vi "SMPS Inversion.vi"(8 "error in (no error)":errorcluster, 11 "DMA in":refnum<class "DMA.lvclass">) -> (0 "error out":errorcluster, 2 "IV Out":sgl[](array[numeric]), 3 "DMA out":refnum<class "DMA.lvclass">)   [LabVIEW 2014, in "DMA.lvclass"]
uses:
  DMA.lvclass
  DMA.lvclass/DMA.ctl
panel:
  out "Finished?":bool
  in  "smooth":u8
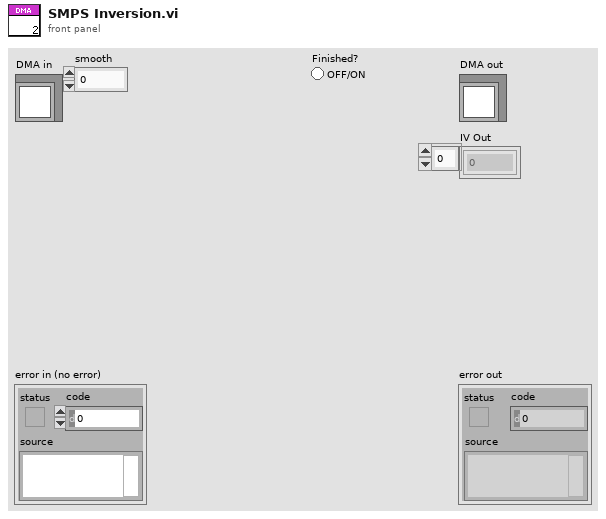
[diagram p1: front panel]
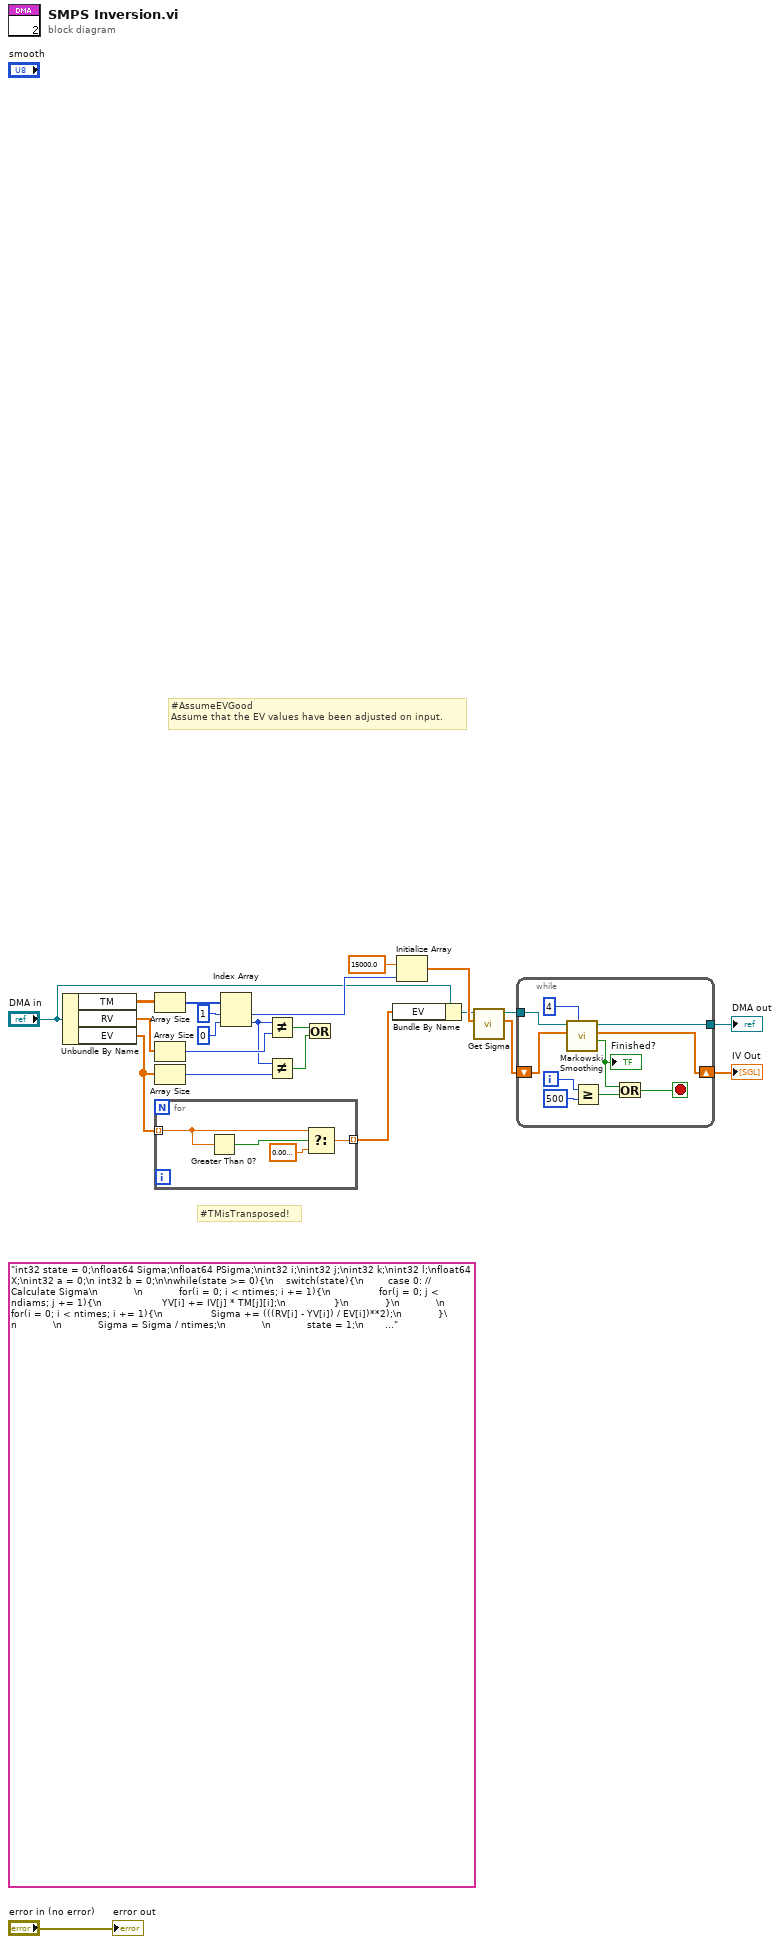
[diagram p0: block diagram]
diagram:
  (unwired) "int32 state = 0;\nfloat64 Sigma;\nfloat64 PSigma;\nint32 i;\nint32 j;\nint32 k;\nint32 l;\nfloat64 X;\nint32 a = 0;\n int32 b = 0;\n\nwhile(state >= 0){\n    switch(state){\n        case 0: // Calculate Sigma\n            \n            for(i = 0; i < ntimes; i += 1){\n                for(j = 0; j < ndiams; j += 1){\n                    YV[i] += IV[j] * TM[j][i];\n                }\n            }\n            \n            for(i = 0; i < ntimes; i += 1){\n                Sigma += (((RV[i] - YV[i]) / EV[i])**2);\n            }\n            \n            Sigma = Sigma / ntimes;\n            \n            state = 1;\n            \n    break;\n        case 1: // Twomey Iterations\n            \n            for(i = 0; i < ntimes; i += 1){\n                for(k = 0; k < ndiams; k += 1){\n                    X += TM[k][i] * IV[k];\n                }\n                X = RV[i] / X;\n                for(j = 0; j < ndiams; j += 1){\n                    IV[j] = (1 + (X - 1) * TM[j][i]) * IV[j];\n                }\n            }\n            \n            PSigma = Sigma;\n\n            for(i = 0; i < ntimes; i += 1){\n                for(j = 0; j < ndiams; j += 1){\n                    YV[i] += IV[j] * TM[j][i];\n                }\n            }\n            \n            for(i = 0; i < ntimes; i += 1){\n                Sigma += (((RV[i] - YV[i]) / EV[i])**2);\n            }\n            \n            Sigma = Sigma / ntimes;\n\n            a += 1;\n            \n            if(a >= 100){state = 2;}\n            \n    break;\n        case 2: // Smoothing\n            \n            for(j = 0; j < ndiams; j += 1){\n                OIV[j] = IV[j];\n            }\n            for(i = 1; i < (ndiams - 2); i += 1){\n                IV[i] = OIV[i - 1] / 4 + OIV[i] / 2 + OIV[i + 1] / 4;\n            }\n            IV[0] = OIV[0] * 3/4 + OIV[1] * 1/4;\n            IV[ndiams - 1] = OIV[ndiams - 1] * 3/4 + OIV[ndiams - 2] * 1/4;\n            \n            b += 1;\n            \n            if(b >= 3){state = -1;}\n            \n    break;\n    }\n}"
  # "#TMisTransposed!"
  # "#AssumeEVGood\nAssume that the EV values have been adjusted on input."
  # "//Test for Errors in Matrix and Vector Dimensions\nint32 Error = 0;\nint32 ntimes;\nint32 ndiams;\nint32 i = 0;\n\nif(sizeOfDim(TM, 1) != sizeOfDim(RV, 0)){\nError = Error + 1;                                     }\nif(sizeOfDim(TM, 1) != sizeOfDim(EV, 0)){\nError = Error + 2;                                     }\nntimes =  sizeOfDim(TM, 1);\nndiams =  sizeOfDim(TM, 0);\n\nfor(i = 0; i < ntimes; i+=1){\n    if(EV[i] == 0 ){ EV[i] = 0.001;}\n    }"
  n1 = Unbundle By Name("DMA in") -> ("TM"=w16:sgl[][], "RV"=w15:sgl[], "EV"=w5:sgl[])
  n2 = Array Size(array=w16) -> (size(s)=w21:i32[])
  n3 = Array Size(array=w15) -> (size(s)=w20:i32)
  n4 = Array Size(array=w5) -> (size(s)=w19:i32)
  n5 = for {
    tunnel: w5 -> [w26] mode=indexing
    tunnel: [w23] -> w3 mode=indexing
    n6 = Greater Than 0?(x=w26) -> (x > 0?=w24:bool)
    n7 = Select(t=w26, s=w24, f=sgl 0.01) -> (s? t:f=w23:sgl)
  }
  n8 = Index Array(array=w21, index #1=1 ("index"), index #2=0 ("index")) -> (element #1=w14:i32, element #2=w11:i32)
  n9 = Not Equal?(x=w11, y=w20) -> (x != y?=w17:bool)
  n10 = Not Equal?(x=w11, y=w19) -> (x != y?=w18:bool)
  n11 = Or(x=w17, y=w18) -> ()  [unwired: 1 out]
  n12 = Bundle By Name(cluster="DMA in", "EV"=w3) -> (w2:refnum<class "DMA.lvclass">)
  n13 = Initialize Array(sgl 15000.0 ("element"), w14) -> (w12:sgl[])
  n14 = call "Get Sigma.vi"("IV in"=w12, "DMA in"=w2) -> ("IV Out"=w7:sgl[], "DMA Out"=w8:refnum<class "DMA.lvclass">)  [unwired: 6 in, 2 out]
  n15 = while {
    tunnel: w8 -> [w36]
    shift-right: [w34] -> w6
    shift-left: w7 -> [w35]
    tunnel: [w32] -> w1
    i -> [w30]
    stop <- w27 stop-if-true
    n16 = call "Markowski Smoothing.vi"("smooth"=u8 4, "IV in"=w35, "DMA in"=w36) -> ("Finished?"=w31:bool, "IV Out"=w34:sgl[], "DMA Out"=w32:refnum<class "DMA.lvclass">)  [unwired: 6 in]
    "Finished?" <- w31
    n17 = Greater Or Equal?(x=w30, y=500) -> (x >= y?=w28:bool)
    n18 = Or(x=w31, y=w28) -> (x .or. y?=w27:bool)
  }
  "DMA out" <- w1
  "IV Out" <- w6
  "error out" <- "error in (no error)"
